vi "Response.vi"(8 "error in (no error)":errorcluster, 11 "Node Ptr":T2 format="%.0x") -> (0 "error out":errorcluster)   [LabVIEW 2019, in "Instrument Addon System Explorer.lvlib"]
uses:
  Instrument Addon System Explorer.lvlib
  <vilib>/NI VeriStand/Custom Device API/Custom Device Item Ref.ctl
  Shared/Types/Response Wait Type.ctl
  NationalInstruments.VeriStand.SystemStorageUI
  Shared/Types/FG Control.ctl
  NationalInstruments.VeriStand.SystemStorage
  Shared/Constants.vi
  <vilib>/NI VeriStand/Custom Device API/NI VeriStand - Get Item Property.vi
  <vilib>/NI VeriStand/Custom Device API/Get Item Property (String).vi
  <vilib>/NI VeriStand/Custom Device API/Get Item Property (String Array).vi
  <vilib>/NI VeriStand/Custom Device API/Get Item Property (Double).vi
  <vilib>/NI VeriStand/Custom Device API/Get Item Property (U32).vi
  <vilib>/NI VeriStand/Custom Device API/Get Item Property (Boolean).vi
  <vilib>/NI VeriStand/Custom Device API/NI VeriStand - Set Item Property.vi
  <vilib>/NI VeriStand/Custom Device API/Set Item Property (String).vi
  <vilib>/NI VeriStand/Custom Device API/Set Item Property (String Array).vi
  <vilib>/NI VeriStand/Custom Device API/Set Item Property (Double).vi
  <vilib>/NI VeriStand/Custom Device API/Set Item Property (U32).vi
  <vilib>/NI VeriStand/Custom Device API/Set Item Property (Boolean).vi
  <vilib>/NI VeriStand/Custom Device API/Custom Device API.lvlib
  Shared/Instrument Addon Shared.lvlib
  <vilib>/NI VeriStand/UI Controls/Single Node Browser/NI_VS UI Single Node Browser.lvlib
panel:
  in  "Channel":refnum<k24>(container) caption="Value"
  in  "Use Channel?":bool
  in  "Linkages":i32(listbox)
  in  "MetaData":string(combo) caption="Available MetaData Channels"
  in  "Response":string caption="Response Format ( Use [] to define a variable )"
  in  "Header 2":cluster{"Section Name":string}={"Section Name"="Response Settings"}
  in  "Wait Type":T1
  in  "Type Value":dbl=100.0 caption="Byte Count Value" format="%#_p"
  in  "SHDocVw.IWebBrowser":refnum<k7>(container)
  in  "Header":cluster{"Section Name":string}={"Section Name"="Custom Device Item Settings"}
  in  "Description":string
  out "Name":string
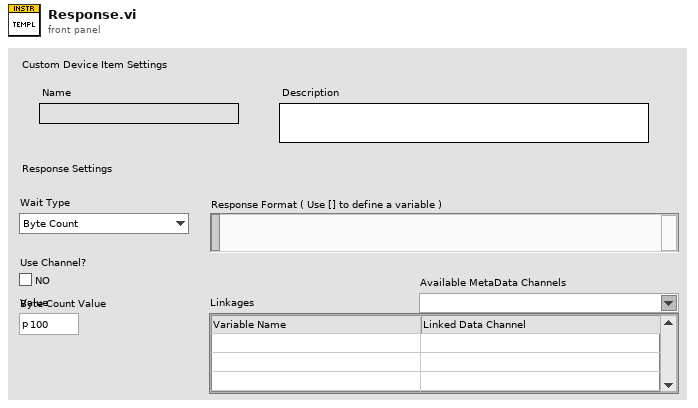
[diagram p1: front panel]
types:
  T1 = typedef "Instrument Addon Shared.lvlib/Response Wait Type.ctl" = enum16{"Byte Count", "Wait sec"}
  T2 = typedef "Custom Device API.lvlib/Custom Device Item Ref.ctl" = u64
  T3 = typedef "Instrument Addon Shared.lvlib/FG Control.ctl" = enum16{"Get", "Set"}
  T4 = typedef "Instrument Addon Shared.lvlib/Response Parameters.ctl" = cluster{"Response":string, "Linked Channels":T5[], "Type Value":dbl, "Wait Type":T1, "Use Channel":bool, "Channel Path":string}
  T5 = typedef "Instrument Addon Shared.lvlib/Linked Channel Cluster.ctl" = cluster{"Variable Name":string, "GUID":string}
  T6 = typedef "Custom Device API.lvlib/Custom Device Item Info.ctl" = cluster{"Name":string, "Is Channel":bool, "GUID":string, "Is Waveform":bool}
  T7 = typedef "Custom Device API.lvlib/Custom Device Commands.ctl" = enum16{"Default", "Item renamed", "Shutdown", "Dynamic button pressed"}
  T8 = typedef "NI_VS UI Single Node Browser.lvlib/Node Ref.ctl" = refnum<k24>
  T9 = typedef "Custom Device API.lvlib/Custom Device Pointer.ctl" = refnum<k24>
  T10 = typedef "LVComboBoxStrsAndValuesArrayTypeDef.ctl" = cluster{"String":string, "Value":string}[]
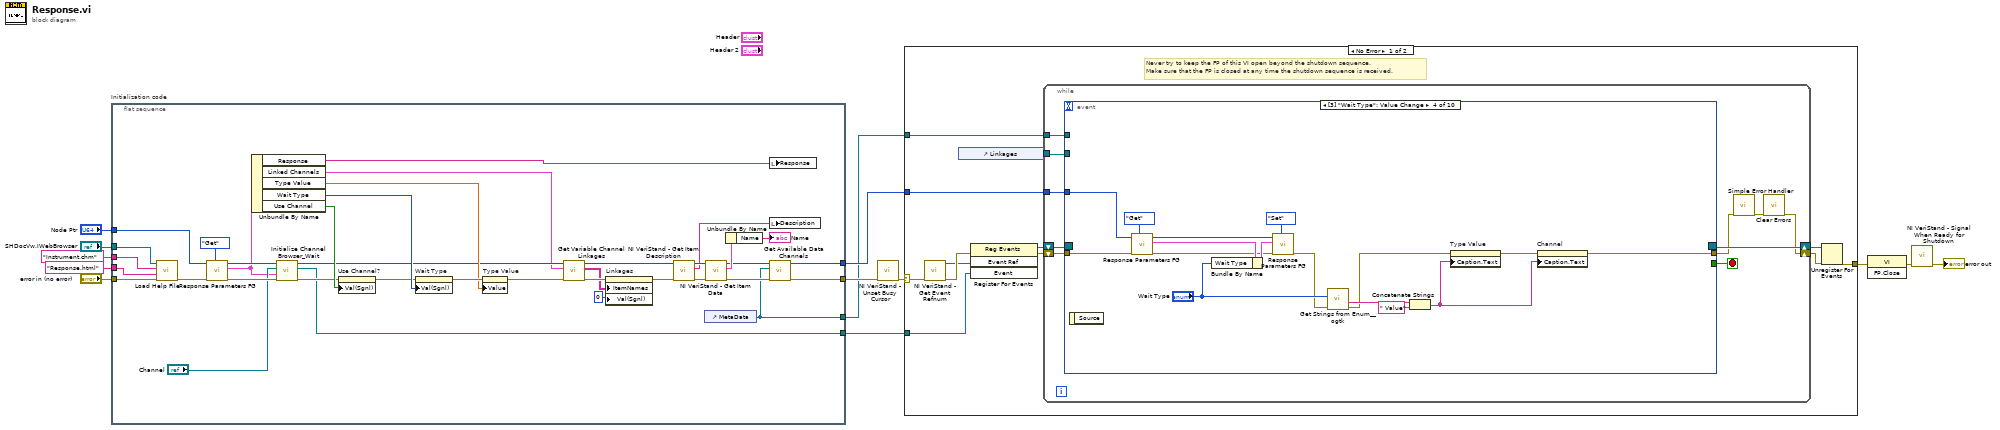
[diagram p0: block diagram]
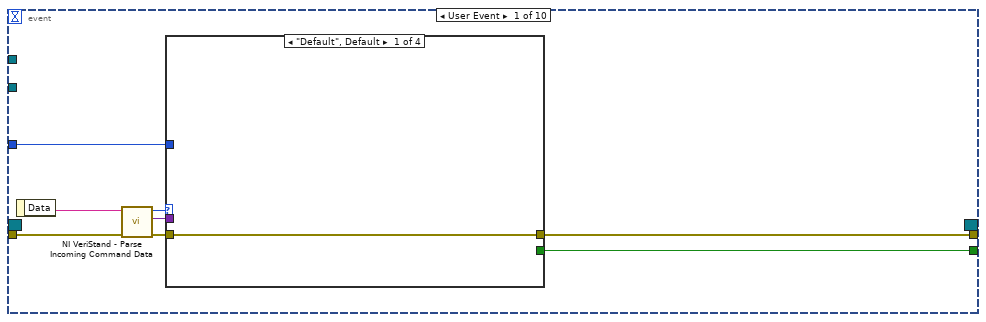
[diagram p2: hidden frame]
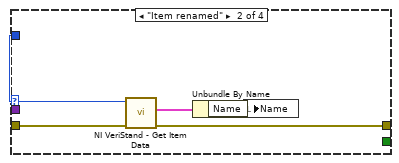
[diagram p3: hidden frame]
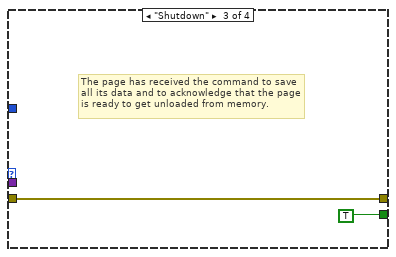
[diagram p4: hidden frame]
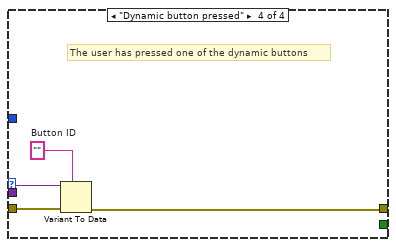
[diagram p5: hidden frame]
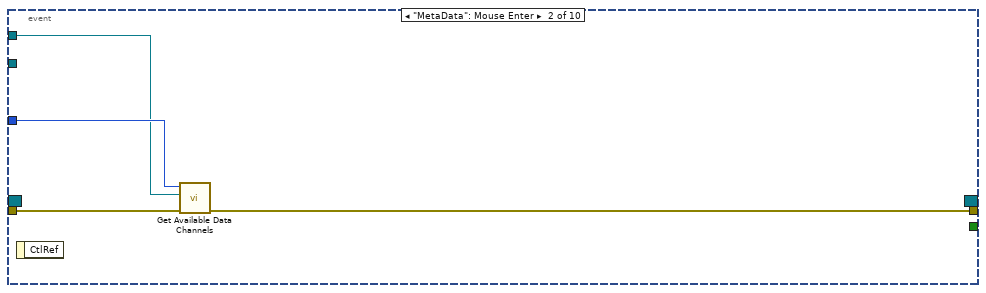
[diagram p6: hidden frame]
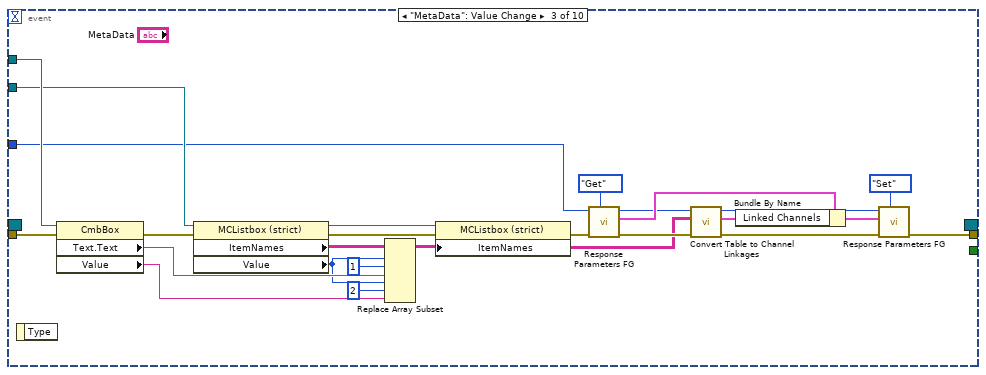
[diagram p7: hidden frame]
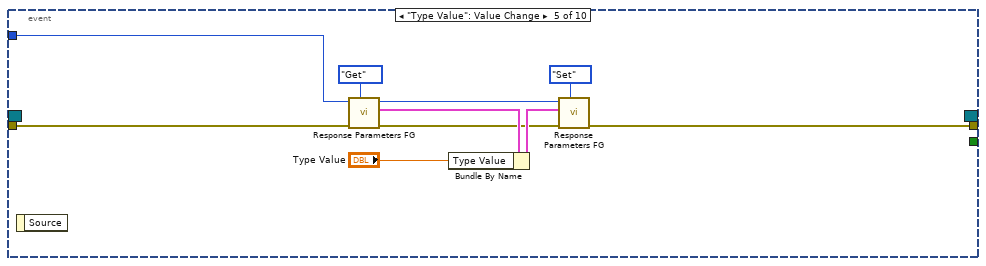
[diagram p8: hidden frame]
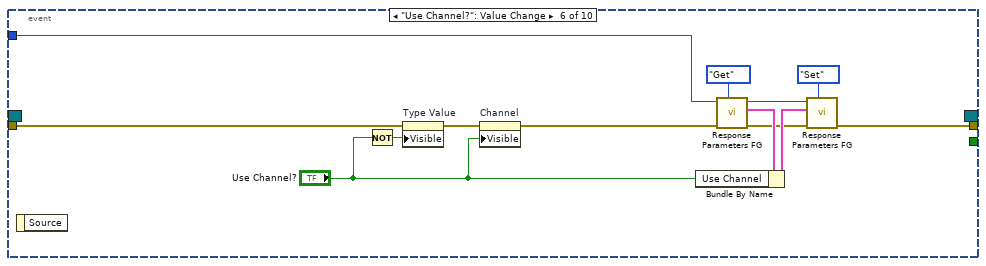
[diagram p9: hidden frame]
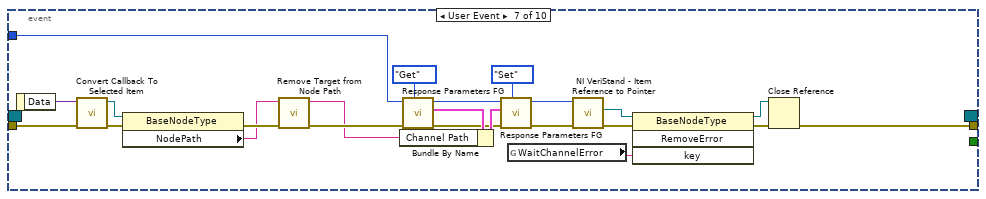
[diagram p10: hidden frame]
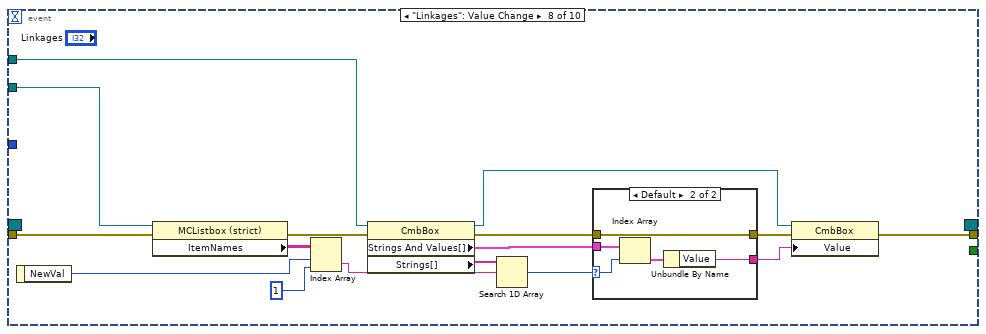
[diagram p11: hidden frame]
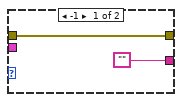
[diagram p12: hidden frame]
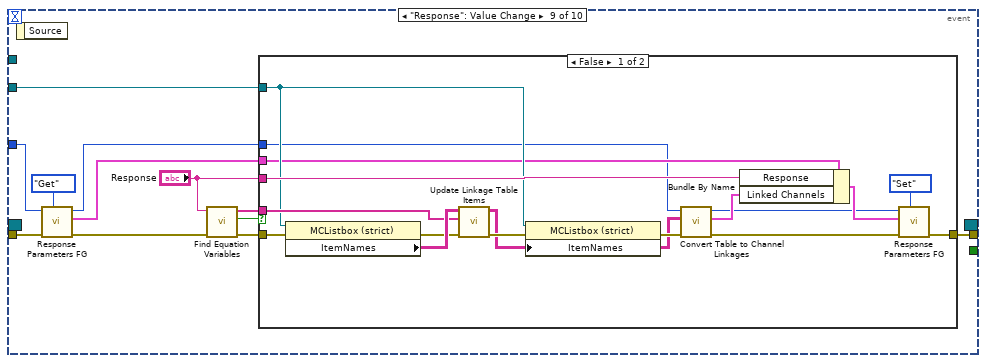
[diagram p13: hidden frame]
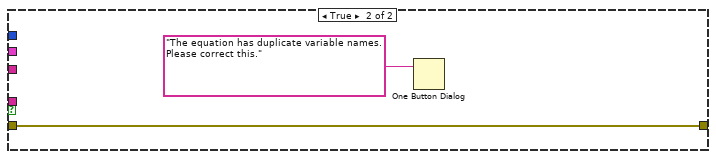
[diagram p14: hidden frame]
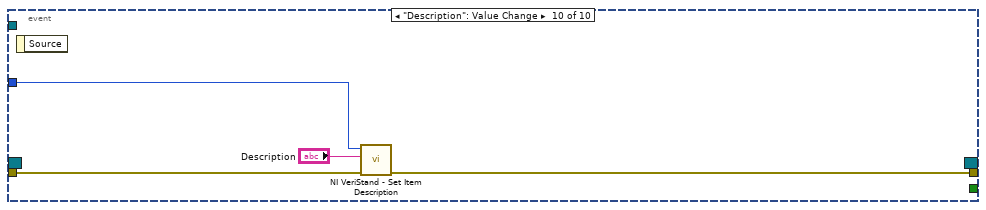
[diagram p15: hidden frame]
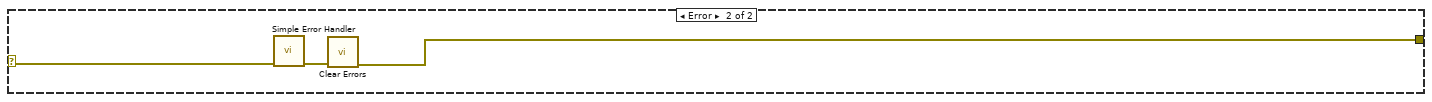
[diagram p16: hidden frame]
diagram:
  n1 = flat-sequence "Initialization code" {
    tunnel: "error in (no error)" -> [w45]
    tunnel: "Node Ptr" -> [w40]
    tunnel: [w34] -> w9
    tunnel: [w32] -> w6
    tunnel: "SHDocVw.IWebBrowser" -> [w44]
    tunnel: "Response.html" ("HTML File") -> [w43]
    tunnel: "Instrument.chm" ("Main CHM File") -> [w42]
    tunnel: [w31] -> w2
    tunnel: [w17] -> w1
    frame #0 {
      n2 = call "Load Help File.vi"("error in (no error)"=w45, "HTML File"=w43, "Main CHM File"=w42, "SHDocVw.IWebBrowser2"=w44) -> ("error out"=w41:errorcluster)  [unwired: 7 in]
      n3 = call "Response Parameters FG.vi"("Action"=FG_Control."Get", "error in (no error)"=w41, "Item Ref in"=w40) -> ("error out"=w21:errorcluster, "Reponse Parameters"=w14:T4, "Item Ref out"=w19:T2)  [unwired: 6 in]
      n4 = Unbundle By Name(w14) -> ("Response"=w36:string, "Linked Channels"=w15:T5[], "Type Value"=w22:dbl, "Wait Type"=w30:T1, "Use Channel"=w23:bool)
      n5 = call "Initialize Channel Browser_Wait.vi"("error in (no error)"=w21, "Reponse Parameters"=w14, ".NET Refnum in"="Channel", "Item Ref in"=w19) -> ("error out"=w20:errorcluster, "Event"=w17:refnum<user-event>, "Item Ref out"=w16:T2)  [unwired: 5 in]
      n6 = property on="Use Channel?" class="Bool (strict)"(error in=w20, "Val(Sgnl)"=w23) -> (error out=w24:errorcluster)  [unwired: 1 in, 1 out]
      n7 = property on="Wait Type" class="Enum (strict)"(error in=w24, "Val(Sgnl)"=w30) -> (error out=w26:errorcluster)  [unwired: 1 in, 1 out]
      n8 = property on="Type Value" class="DigNum (strict)"(error in=w26, "Value"=w22) -> (error out=w25:errorcluster)  [unwired: 1 in, 1 out]
      n9 = call "Get Variable Channel Linkages.vi"("error in (no error)"=w25, "Linked Channels"=w15, "Item Ref in"=w16) -> ("error out"=w29:errorcluster, "Array"=w27:string[][], "Item Ref out"=w28:T2)  [unwired: 6 in]
      n10 = property on="Linkages" class="MCListbox (strict)"(error in=w29, "ItemNames"=w27, "Val(Sgnl)"=0 ("Value (Signaling)")) -> (error out=w37:errorcluster)  [unwired: 1 in, 1 out]
      n11 = call <vilib>:"NI VeriStand - Get Item Description.vi"("error in (no error)"=w37, "Item Ref in"=w28) -> ("error out"=w48:errorcluster, "Description"=w49:string, "Item Ref out"=w50:T2)  [unwired: 7 out]
      n12 = control-ref of="MetaData"() -> (w31:refnum<vi>)
      n13 = call <vilib>:"NI VeriStand - Get Item Data.vi"("error in (no error)"=w48, "Item Ref in"=w50) -> ("error out"=w35:errorcluster, "Item Info"=w47:T6, "Item Ref out"=w33:T2)  [unwired: 7 out]
      n14 = Unbundle By Name(w47) -> ("Name"=→"Name":string)
      n15 = local write "Response"(w36) -> ()
      n16 = local write "Description"(w49) -> ()
      n17 = call "Get Available Data Channels.vi"("error in (no error)"=w35, "MetaData"=w31, "Item Ref in"=w33) -> ("error out"=w34:errorcluster, "Item Ref out"=w32:T2)  [unwired: 7 in]
    }
  }
  n18 = call <vilib>:"NI VeriStand - Unset Busy Cursor.vi"("error in (no error)"=w9) -> ("error out"=w8:errorcluster)  [unwired: 10 out]
  n19 = case shown="No Error" w8 {
    selector: w8 -> [w54 w244]
    tunnel: [w59 w242] -> w13
    tunnel: w6 -> [w55 _]
    tunnel: w2 -> [w52 _]
    tunnel: w1 -> [w51 _]
    frame No Error {
      # "Never try to keep the FP of this VI open beyond the shutdown sequence.\nMake sure that the FP is closed at any time the shutdown sequence is received."
      n20 = call <vilib>:"NI VeriStand - Get Event Refnum.vi"("error in (no error)"=w54) -> ("error out"=w62:errorcluster, "Event Ref"=w58:refnum<user-event>)  [unwired: 9 out]
      n21 = control-ref of="Linkages"() -> (w53:refnum<vi>)
      n22 = register-events(error in=w62, w58, w51) -> (reference out=w56:refnum<event-registration>, error out=w57:errorcluster)  [unwired: 1 in]
      n23 = while {
        tunnel: w55 -> [w68]
        shift-right: [w65] -> w60
        shift-left: w57 -> [w71]
        shift-right: [w72] -> w61
        shift-left: w56 -> [w70]
        tunnel: w53 -> [w63]
        tunnel: w52 -> [w64]
        stop <- w69 stop-if-true
        n24 = event shown="[3] \"Wait Type\": Value Change" {
          selector: w70 -> [_ _ _ _ _ _ _ _ _ _]
          dyn-events: [_ _ _ _ _ _ _ _ _ _] -> w72
          timeout: _ -> [_ _ _ _ _ _ _ _ _ _]
          tunnel: w71 -> [w80 w96 w106 w131 w141 w159 w181 w188 w212 w240]
          tunnel: [w76 _ _ _ _ _ _ _ _ _] -> w69
          tunnel: [w75 w93 w102 w123 w138 w150 w163 w184 w215 w239] -> w67
          tunnel: w68 -> [w74 w95 w103 w132 w142 w148 w173 _ w210 w241]
          tunnel: w64 -> [_ w94 w105 _ _ _ _ w187 _ _]
          tunnel: w63 -> [_ _ w104 _ _ _ _ w186 w214 _]
          event User Event {
            n25 = event-data() -> ("Data"=w79:string)  [unwired: 1 out]
            n26 = call <vilib>:"NI VeriStand - Parse Incoming Command Data.vi"("error in (no error)"=w80, "Incoming data"=w79) -> ("error out"=w78:errorcluster, "Outgoing data"=w73:variant, "Action"=w77:T7)  [unwired: 7 out]
            n27 = case shown="\"Default\", Default" w77 {
              tunnel: w78 -> [w81 w86 w87 w92]
              tunnel: [_ _ TRUE _] -> w76
              tunnel: [w81 w83 w87 w89] -> w75
              tunnel: w74 -> [_ w85 _ _]
              tunnel: w73 -> [_ _ _ w91]
              frame "Default", Default {
              }
              frame "Item renamed" {
                n28 = call <vilib>:"NI VeriStand - Get Item Data.vi"("error in (no error)"=w86, "Item Ref in"=w85) -> ("error out"=w83:errorcluster, "Item Info"=w84:T6)  [unwired: 8 out]
                n29 = Unbundle By Name(w84) -> ("Name"=w82:string)
                n30 = local write "Name"(w82) -> ()
              }
              frame "Shutdown" {
                # "The page has received the command to save all its data and to acknowledge that the page is ready to get unloaded from memory."
              }
              frame "Dynamic button pressed" {
                w90 = ""  # Button ID
                # "The user has pressed one of the dynamic buttons"
                n31 = Variant To Data(error in=w92, type=w90, Variant=w91) -> (error out=w89:errorcluster)  [unwired: 1 out]
              }
            }
          }
          event "MetaData": Mouse Enter {
            n32 = event-data() -> ()  [unwired: 2 out]
            n33 = call "Get Available Data Channels.vi"("error in (no error)"=w96, "MetaData"=w94, "Item Ref in"=w95) -> ("error out"=w93:errorcluster)  [unwired: 7 in, 1 out]
          }
          event "MetaData": Value Change {
            n34 = event-data() -> ()  [unwired: 2 out]
            n35 = property class="CmbBox"(reference=w105, error in=w106) -> (error out=w109:errorcluster, "Text.Text"=w108:string, "Value"=w101:string)  [unwired: 1 out]
            n36 = property class="MCListbox (strict)"(reference=w104, error in=w109) -> (reference out=w119:refnum<vi>, error out=w118:errorcluster, "ItemNames"=w121:string[][], "Value"=w107:i32)
            n37 = Replace Array Subset(array=w121, new element #1=w108, index (row) #1=w107, index (col) #1=1 ("disabled index (col)"), new element #2=w101, index (row) #2=w107, index (col) #2=2 ("disabled index (col)")) -> (w100:string[][])
            n38 = property class="MCListbox (strict)"(reference=w119, error in=w118, "ItemNames"=w100) -> (error out=w113:errorcluster)  [unwired: 1 out]
            n39 = call "Response Parameters FG.vi"("Action"=FG_Control."Get", "error in (no error)"=w113, "Item Ref in"=w103) -> ("error out"=w112:errorcluster, "Reponse Parameters"=w111:T4, "Item Ref out"=w98:T2)  [unwired: 6 in]
            n40 = call "Convert Table to Channel Linkages.vi"("error in (no error)"=w112, "Item Names"=w100, "Item Ref in"=w98) -> ("error out"=w116:errorcluster, "Linkages"=w99:T5[], "Item Ref out"=w97:T2)  [unwired: 6 in]
            n41 = Bundle By Name(cluster=w111, "Linked Channels"=w99) -> (w115:T4)
            n42 = call "Response Parameters FG.vi"("Action"=FG_Control."Set", "error in (no error)"=w116, "Reponse Parameters"=w115, "Item Ref in"=w97) -> ("error out"=w102:errorcluster)  [unwired: 5 in, 2 out]
          }
          event Value Change {
            n43 = event-data() -> ()  [unwired: 2 out]
            n44 = call "Response Parameters FG.vi"("Action"=FG_Control."Get", "error in (no error)"=w131, "Item Ref in"=w132) -> ("error out"=w130:errorcluster, "Reponse Parameters"=w134:T4, "Item Ref out"=w133:T2)  [unwired: 6 in]
            n45 = Bundle By Name(cluster=w134, "Wait Type"="Wait Type") -> (w136:T4)
            n46 = call "Response Parameters FG.vi"("Action"=FG_Control."Set", "error in (no error)"=w130, "Reponse Parameters"=w136, "Item Ref in"=w133) -> ("error out"=w127:errorcluster)  [unwired: 5 in, 2 out]
            n47 = call <userlib>:"Get Strings from Enum__ogtk.vi"("error in (no error)"=w127, "Enum"="Wait Type") -> ("error out"=w126:errorcluster, "String Value"=w128:string)  [unwired: 6 in, 2 out]
            n48 = Concatenate Strings(w128, " Value" ("string")) -> (w122:string)
            n49 = property on="Type Value" class="DigNum (strict)"(error in=w126, "Caption.Text"=w122) -> (error out=w124:errorcluster)  [unwired: 1 in, 1 out]
            n50 = property on="Channel" class="AXCont"(error in=w124, "Caption.Text"=w122) -> (error out=w123:errorcluster)  [unwired: 1 in, 1 out]
          }
          event "Type Value": Value Change {
            n51 = event-data() -> ()  [unwired: 2 out]
            n52 = call "Response Parameters FG.vi"("Action"=FG_Control."Get", "error in (no error)"=w141, "Item Ref in"=w142) -> ("error out"=w140:errorcluster, "Reponse Parameters"=w144:T4, "Item Ref out"=w143:T2)  [unwired: 6 in]
            n53 = Bundle By Name(cluster=w144, "Type Value"="Type Value") -> (w146:T4)
            n54 = call "Response Parameters FG.vi"("Action"=FG_Control."Set", "error in (no error)"=w140, "Reponse Parameters"=w146, "Item Ref in"=w143) -> ("error out"=w138:errorcluster)  [unwired: 5 in, 2 out]
          }
          event "Use Channel?": Value Change {
            n55 = event-data() -> ()  [unwired: 2 out]
            n56 = Not(x="Use Channel?") -> (.not. x?=w158:bool)
            n57 = property on="Type Value" class="DigNum (strict)"(error in=w159, "Visible"=w158) -> (error out=w160:errorcluster)  [unwired: 1 in, 1 out]
            n58 = property on="Channel" class="AXCont"(error in=w160, "Visible"="Use Channel?") -> (error out=w151:errorcluster)  [unwired: 1 in, 1 out]
            n59 = call "Response Parameters FG.vi"("Action"=FG_Control."Get", "error in (no error)"=w151, "Item Ref in"=w148) -> ("error out"=w152:errorcluster, "Reponse Parameters"=w154:T4, "Item Ref out"=w153:T2)  [unwired: 6 in]
            n60 = Bundle By Name(cluster=w154, "Use Channel"="Use Channel?") -> (w156:T4)
            n61 = call "Response Parameters FG.vi"("Action"=FG_Control."Set", "error in (no error)"=w152, "Reponse Parameters"=w156, "Item Ref in"=w153) -> ("error out"=w150:errorcluster)  [unwired: 5 in, 2 out]
          }
          event User Event {
            n62 = event-data() -> ("Data"=w180:variant)  [unwired: 1 out]
            n63 = call <vilib>:"Convert Callback To Selected Item.vi"("error in"=w181, "Data"=w180) -> ("error out"=w182:errorcluster, "Selected Item"=w183:T8)  [unwired: 8 in]
            n64 = property class="BaseNodeType"(reference=w183, error in=w182) -> (error out=w172:errorcluster, "NodePath"=w171:string)  [unwired: 1 out]
            n65 = call "Remove Target from Node Path.vi"("error in (no error)"=w172, "NodePath"=w171) -> ("error out"=w170:errorcluster, "PathArrayToString"=w169:string)  [unwired: 8 in]
            n66 = call "Response Parameters FG.vi"("Action"=FG_Control."Get", "error in (no error)"=w170, "Item Ref in"=w173) -> ("error out"=w174:errorcluster, "Reponse Parameters"=w176:T4, "Item Ref out"=w175:T2)  [unwired: 6 in]
            n67 = Bundle By Name(cluster=w176, "Channel Path"=w169) -> (w178:T4)
            n68 = call "Response Parameters FG.vi"("Action"=FG_Control."Set", "error in (no error)"=w174, "Reponse Parameters"=w178, "Item Ref in"=w175) -> ("error out"=w164:errorcluster, "Item Ref out"=w162:T2)  [unwired: 5 in, 1 out]
            n69 = global read "Constants.vi" "WaitChannelError"() -> (w161:string)
            n70 = call <vilib>:"NI VeriStand - Item Reference to Pointer.vi"("error in (no error)"=w164, "Item Ref in"=w162) -> ("error out"=w166:errorcluster, "Node Pointer"=w165:T9)  [unwired: 6 in, 2 out]
            n71 = invoke class="BaseNodeType" method="RemoveError"(reference=w165, error in=w166, "key"=w161) -> (reference out=w168:T9, error out=w167:errorcluster)  [unwired: 1 in, 2 out]
            n72 = Close Reference(reference=w168, error in (no error)=w167) -> (error out=w163:errorcluster)
          }
          event "Linkages": Value Change {
            n73 = event-data() -> ("NewVal"=w185:i32)  [unwired: 1 out]
            n74 = property class="MCListbox (strict)"(reference=w186, error in=w188) -> (error out=w197:errorcluster, "ItemNames"=w199:string[][])  [unwired: 1 out]
            n75 = Index Array(array=w199, index (row)=w185, index (col)=1 ("disabled index (col)")) -> (element=w196:string)
            n76 = property class="CmbBox"(reference=w187, error in=w197) -> (reference out=w192:refnum<vi>, error out=w190:errorcluster, "Strings And Values[]"=w195:T10, "Strings[]"=w189:string[])
            n77 = Search 1D Array(1D array=w189, element=w196) -> (index of element=w193:i32)  [unwired: 1 in]
            n78 = case shown="Default" w193 {
              selector: w193 -> [_ w204]
              tunnel: w195 -> [_ w206]
              tunnel: ["" w202] -> w194
              tunnel: [w201 w203] -> w191
              tunnel: w190 -> [w201 w203]
              frame -1 {
              }
              frame Default {
                n79 = Index Array(array=w206, index=w204) -> (element=w205:cluster{"String":string, "Value":string})
                n80 = Unbundle By Name(w205) -> ("Value"=w202:string)
              }
            }
            n81 = property class="CmbBox"(reference=w192, error in=w191, "Value"=w194) -> (error out=w184:errorcluster)  [unwired: 1 out]
          }
          event "Response": Value Change {
            n82 = event-data() -> ()  [unwired: 2 out]
            n83 = call "Response Parameters FG.vi"("Action"=FG_Control."Get", "error in (no error)"=w212, "Item Ref in"=w210) -> ("error out"=w211:errorcluster, "Reponse Parameters"=w208:T4, "Item Ref out"=w209:T2)  [unwired: 6 in]
            n84 = call "Find Equation Variables.vi"("error in (no error)"=w211, "Command"="Response") -> ("error out"=w218:errorcluster, "Duplicate?"=w207:bool, "Variables"=w217:string[])  [unwired: 7 in]
            n85 = case shown="False" w207 {
              tunnel: w218 -> [w229 w237]
              tunnel: w217 -> [w228 _]
              tunnel: "Response" -> [w227 _]
              tunnel: [w226 w237] -> w215
              tunnel: w214 -> [w225 _]
              tunnel: w209 -> [w220 _]
              tunnel: w208 -> [w224 _]
              frame False {
                n86 = property class="MCListbox (strict)"(reference=w225, error in=w229) -> (error out=w230:errorcluster, "ItemNames"=w231:string[][])  [unwired: 1 out]
                n87 = call "Update Linkage Table Items.vi"("error in (no error)"=w230, "Variables"=w228, "Item Names"=w231) -> ("error out"=w232:errorcluster, "Item Names"=w222:string[][])  [unwired: 7 in]
                n88 = property class="MCListbox (strict)"(reference=w225, error in=w232, "ItemNames"=w222) -> (error out=w234:errorcluster)  [unwired: 1 out]
                n89 = call "Convert Table to Channel Linkages.vi"("error in (no error)"=w234, "Item Names"=w222, "Item Ref in"=w220) -> ("error out"=w235:errorcluster, "Linkages"=w221:T5[], "Item Ref out"=w219:T2)  [unwired: 6 in]
                n90 = Bundle By Name(cluster=w224, "Response"=w227, "Linked Channels"=w221) -> (w223:T4)
                n91 = call "Response Parameters FG.vi"("Action"=FG_Control."Set", "error in (no error)"=w235, "Reponse Parameters"=w223, "Item Ref in"=w219) -> ("error out"=w226:errorcluster)  [unwired: 5 in, 2 out]
              }
              frame True {
                n92 = One Button Dialog(message="The equation has duplicate variable names.  Please correct this.") -> ()  [unwired: 1 in, 1 out]
              }
            }
          }
          event "Description": Value Change {
            n93 = event-data() -> ()  [unwired: 2 out]
            n94 = call <vilib>:"NI VeriStand - Set Item Description.vi"("error in (no error)"=w240, "Description"="Description", "Item Ref in"=w241) -> ("error out"=w239:errorcluster)  [unwired: 8 out]
          }
        }
        n95 = call <vilib>:"Simple Error Handler.vi"("error in (no error)"=w67) -> ("error out"=w66:errorcluster)  [unwired: 1 in, 7 out]
        n96 = call <vilib>:"Clear Errors.vi"("error in (no error)"=w66) -> ("error out"=w65:errorcluster)  [unwired: 1 in, 5 out]
      }
      n97 = Unregister For Events(event registration refnum=w61, error in=w60) -> (error out=w59:errorcluster)
    }
    frame Error {
      n98 = call <vilib>:"Simple Error Handler.vi"("error in (no error)"=w244) -> ("error out"=w243:errorcluster)  [unwired: 1 in, 7 out]
      n99 = call <vilib>:"Clear Errors.vi"("error in (no error)"=w243) -> ("error out"=w242:errorcluster)  [unwired: 1 in, 5 out]
    }
  }
  n100 = invoke class="VI" method="FP.Close"(error in=w13) -> (error out=w12:errorcluster)  [unwired: 2 in, 2 out]
  n101 = call <vilib>:"NI VeriStand - Signal When Ready for Shutdown.vi"("error in (no error)"=w12) -> ("error out"=→"error out":errorcluster)  [unwired: 10 out]
